vi "CRC校验1.vi"(1 "要校验的字符串（十六进制显示）":string) -> (0 "CRC32效验码输出":string)   [LabVIEW 2016, in "TCP文件传输系统.lvlib" / "TCP发送文件.lvlib"]
panel:
  out "输出字符串":string
  in  "停止":bool
  out "CRC校验":bool
  out "PSI/SI表":u8[](array[numeric]) format="%.0x"
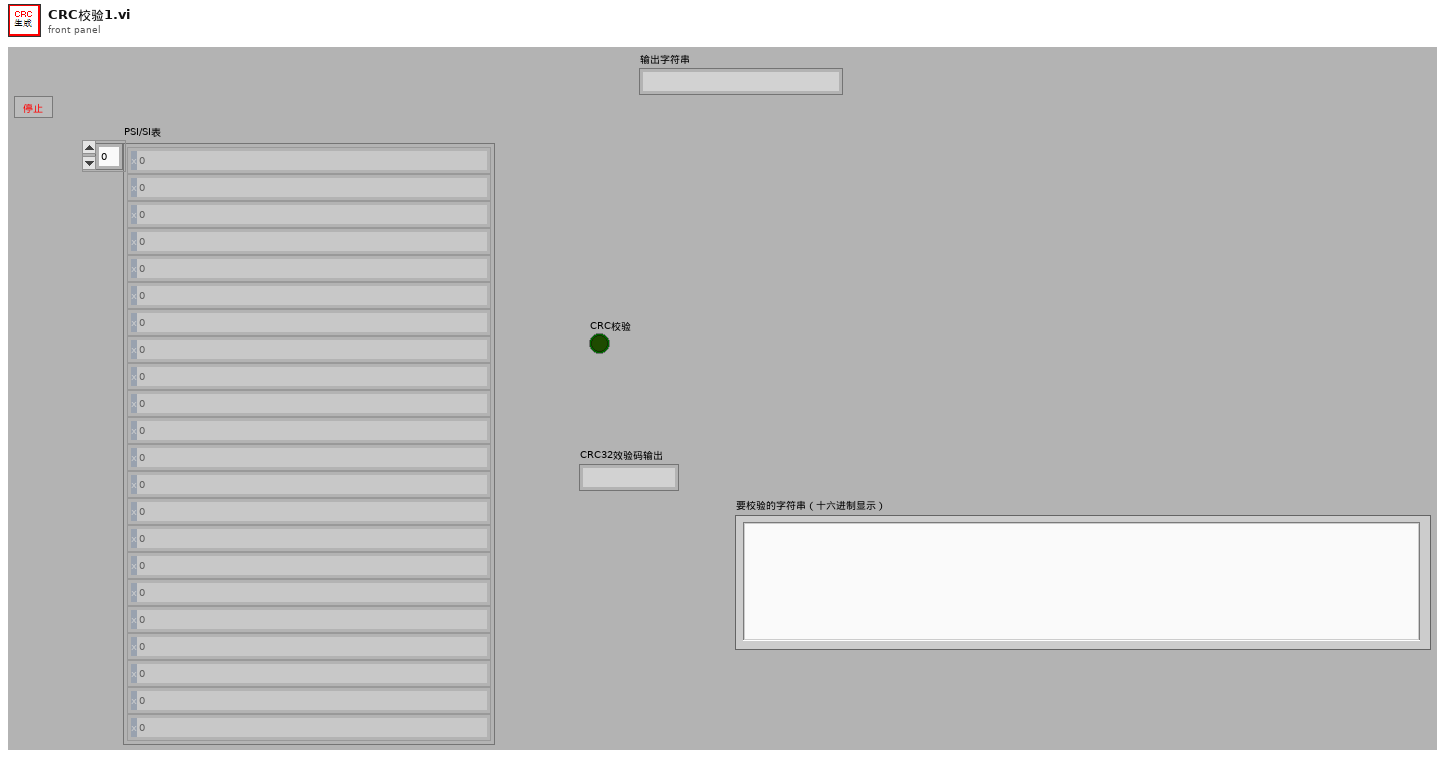
[diagram p1: front panel]
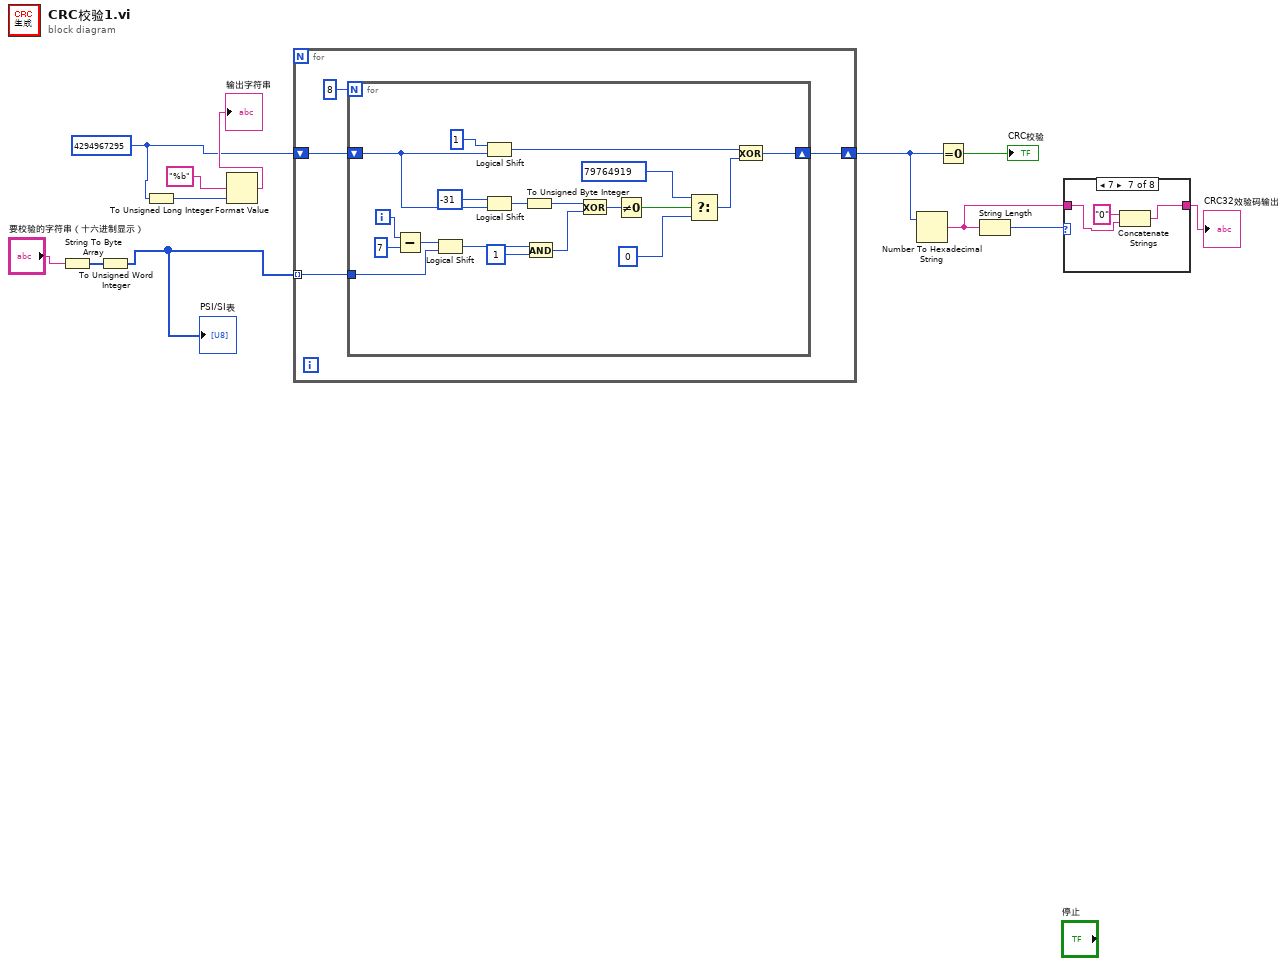
[diagram p0: block diagram]
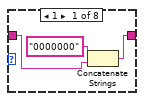
[diagram p2: hidden frame]
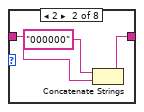
[diagram p3: hidden frame]
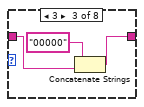
[diagram p4: hidden frame]
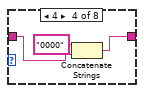
[diagram p5: hidden frame]
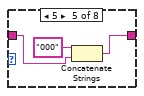
[diagram p6: hidden frame]
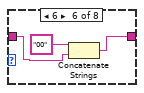
[diagram p7: hidden frame]
diagram:
  w5 = u32 4294967295
  n1 = String To Byte Array(string="要校验的字符串（十六进制显示）") -> (unsigned byte array=w10:u8[])
  n2 = To Unsigned Word Integer(number=w10) -> (unsigned 16bit integer=w8:u16[])
  "PSI/SI表" <- w8
  n3 = To Unsigned Long Integer(number=w5) -> (unsigned 32bit integer=w4:u32)
  n4 = Format Value(format string="%b" ("字符串(\"\")"), value (0)=w4) -> (output string=→"输出字符串":string)  [unwired: 1 in]
  n5 = for {
    tunnel: w8 -> [w16] mode=indexing
    shift-right: [w14] -> w9
    shift-left: w5 -> [w15]
    n6 = for {
      N: 8 -> [_]
      tunnel: w16 -> [w32]
      shift-right: [w34] -> w14
      shift-left: w15 -> [w26]
      i -> [w18]
      n7 = Subtract(x=w18, y=7) -> (x-y=w33:i32)
      n8 = Logical Shift(y=w33, x=w32) -> (x << y=w31:u16)
      n9 = Logical Shift(y=1 ("x"), x=w26) -> (x << y=w35:u32)
      n10 = Logical Shift(y=-31 ("x"), x=w26) -> (x << y=w25:u32)
      n11 = To Unsigned Byte Integer(number=w25) -> (unsigned 8bit integer=w24:u8)
      n12 = And(x=w31, y=u8 1) -> (x .and. y?=w29:u16)
      n13 = Exclusive Or(1:w29, 2:w24) -> (0:w23:u16)
      n14 = Not Equal To 0?(x=w23) -> (x != 0?=w22:bool)
      n15 = Select(t=u32 79764919, s=w22, f=u32 0) -> (s? t:f=w19:u32)
      n16 = Exclusive Or(1:w19, 2:w35) -> (0:w34:u32)
    }
  }
  n17 = Number To Hexadecimal String(2:w9) -> (0:w1:string)  [unwired: 1 in]
  n18 = Equal To 0?(x=w9) -> (x = 0?=→"CRC校验":bool)
  n19 = String Length(string=w1) -> (length=w3:i32)
  n20 = case shown="7" w3 {
    tunnel: [w36 w40 w43 w46 w49 w51 w56 w57] -> w2
    tunnel: w1 -> [w37 w39 w42 w45 w48 w52 w54 w57]
    frame 1 {
      n21 = Concatenate Strings("0000000", w37) -> (w36:string)
    }
    frame 2 {
      n22 = Concatenate Strings("000000", w39) -> (w40:string)
    }
    frame 3 {
      n23 = Concatenate Strings("00000", w42) -> (w43:string)
    }
    frame 4 {
      n24 = Concatenate Strings("0000", w45) -> (w46:string)
    }
    frame 5 {
      n25 = Concatenate Strings("000", w48) -> (w49:string)
    }
    frame 6 {
      n26 = Concatenate Strings("00", w52) -> (w51:string)
    }
    frame 7 {
      n27 = Concatenate Strings("0" ("字符串"), w54) -> (w56:string)
    }
    frame 8, Default {
    }
  }
  "CRC32效验码输出" <- w2
